vi "Gyro Acc Dec Fwd Dis WIND.vi"(4 "Stop rotation":i32=1200, 6 "Ini. Degrees":sgl, 7 "Motor":cluster{"Port":T2, "Port":T2}={"Port"=1, "Port"=2} {"Port" items=["Port A", "Port B", "Port C", "Port D"]; "Port" items=["Port A", "Port B", "Port C", "Port D"]}, 8 "Threshold to De-acc":i32=1000, 9 "De-acc":i32=40, 10 "Acc":i32=80, 11 "EV3 in":T1) -> (3 "EV3 out":T1)   [LabVIEW 2016]
uses:
  <vilib>/NXT/Block Support/NXT_OutputPort.ctl
  <vilib>/NXT/Subs/LVHSConnector.ctl
  <vilib>/NXT/LegoClasses/BrickReference/BrickReference.lvclass
  <vilib>/NXT/Block Support/NXT_InputPort.ctl
  <vilib>/NXT/NXTIO Xnodes/NXTIONodeSubVIs/LEGOResetMotors.vi
  <vilib>/NXT/Dual Mode Library/Motors/Rotation.vi
  <vilib>/NXT/Dual Mode Library/Sensors/EV3_Gyro_Angle.vi
  <vilib>/NXT/NXTIO Xnodes/NXTIONodeSubVIs/NXTMotorSteeringOn.vi
  <vilib>/NXT/NXTIO Xnodes/NXTIONodeSubVIs/NXTStopMotors.vi
  <vilib>/NXT/Dual Mode Library/Waits/Wait_Num.vi
  <vilib>/NXT/NXTIO Xnodes/NXTIOXNode/NXTIO.xnode
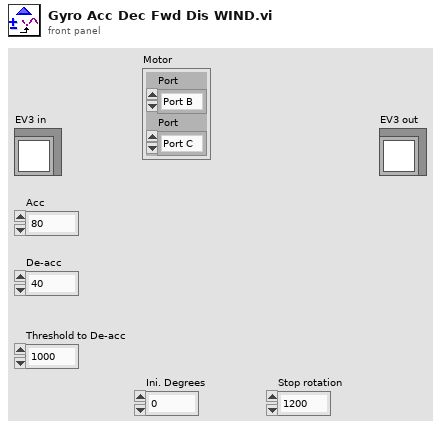
[diagram p1: front panel]
types:
  T1 = typedef "LVHSConnector.ctl" = refnum<class "BrickReference.lvclass">
  T2 = typedef "NXT_OutputPort.ctl" = u8
  T3 = typedef "NXT_InputPort.ctl" = u32
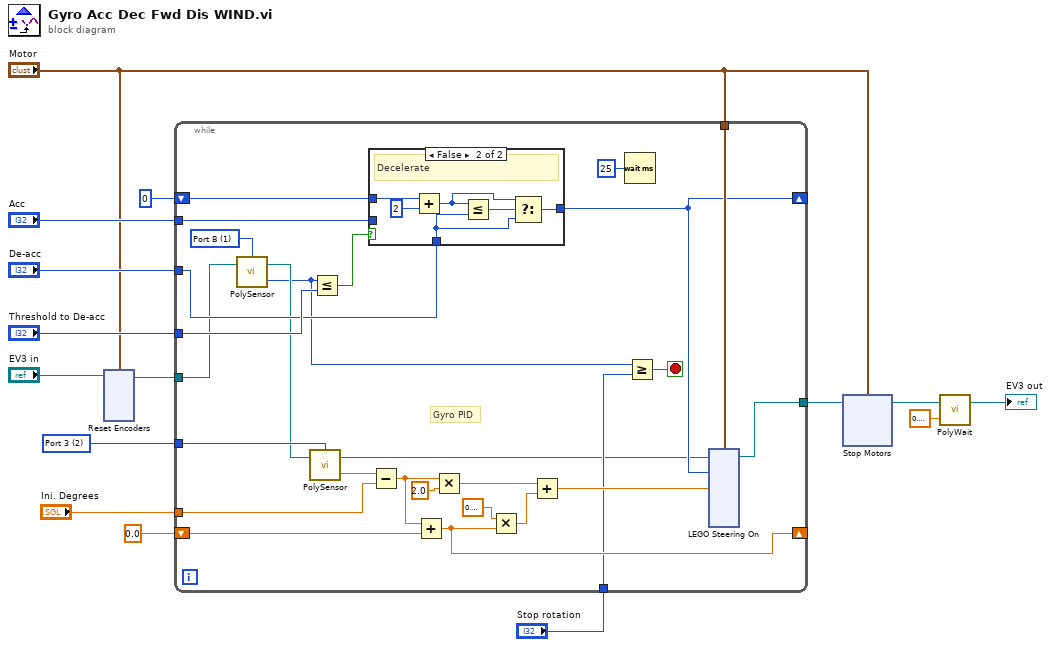
[diagram p0: block diagram]
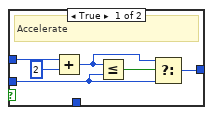
[diagram p2: hidden frame]
diagram:
  w13 = T3 2 items=["Port 1", "Port 2", "Port 3", "Port 4"] ("Port (Gyro)")
  n1 = xnode "Reset Encoders"("Motors"="Motor", "NXT/EV3"="EV3 in") -> ("NXT/EV3"=w10:T1)
  n2 = while {
    tunnel: w10 -> [w23]
    tunnel: w13 -> [w31]
    shift-right: [w39] -> _
    shift-left: sgl 0.0 -> [w40]
    tunnel: "Ini. Degrees" -> [w35]
    tunnel: [w30] -> w6
    tunnel: "Motor" -> [w33]
    shift-right: [w20] -> _
    shift-left: 0 -> [w27]
    tunnel: "De-acc" -> [w24]
    tunnel: "Acc" -> [w26]
    tunnel: "Threshold to De-acc" -> [w25]
    tunnel: "Stop rotation" -> [w17]
    stop <- w19 stop-if-true
    w32 = T2 1 items=["Port A", "Port B", "Port C", "Port D"] ("Port (Port A)")
    # "Gyro PID"
    n3 = call-poly <vilib>:"PolySensor.vi"("NXT/EV3"=w23, "Port (Port A)"=w32) -> ("Angle of Rotation"=w18:i32, "NXT/EV3"=w22:T1)  [unwired: 1 in]
    n4 = call-poly <vilib>:"PolySensor.vi"("NXT/EV3"=w22, "Port (Port 1)"=w31) -> ("Degrees"=w42:sgl, "NXT/EV3"=w16:T1)  [unwired: 1 in]
    n5 = Less Or Equal?(x=w18, y=w25) -> (x <= y?=w21:bool)
    n6 = case shown="False" w21 {
      tunnel: w26 -> [w44 _]
      tunnel: w27 -> [w47 w53]
      tunnel: [w43 w50] -> w20
      tunnel: w24 -> [_ w49]
      frame True {
        # "Accelerate"
        n7 = Add(x=w47, y=2) -> (x+y=w45:i32)
        n8 = Less Or Equal?(x=w45, y=w44) -> (x <= y?=w46:bool)
        n9 = Select(t=w45, s=w46, f=w44) -> (s? t:f=w43:i32)
      }
      frame False {
        # "Decelerate"
        n10 = Add(x=w53, y=2) -> (x+y=w51:i32)
        n11 = Less Or Equal?(x=w51, y=w49) -> (x <= y?=w52:bool)
        n12 = Select(t=w51, s=w52, f=w49) -> (s? t:f=w50:i32)
      }
    }
    n13 = Subtract(x=w42, y=w35) -> (x-y=w34:sgl)
    n14 = Add(x=w34, y=w40) -> (x+y=w39:sgl)
    n15 = Multiply(x=w34, y=sgl 2.0 ("K_p")) -> (x*y=w37:sgl)
    n16 = Multiply(x=sgl 0.1 ("K_i"), y=w39) -> (x*y=w36:sgl)
    n17 = Add(x=w37, y=w36) -> (x+y=w28:sgl)
    n18 = Wait (ms)(milliseconds to wait=u32 25) -> ()  [unwired: 1 out]
    n19 = Greater Or Equal?(x=w18, y=w17) -> (x >= y?=w19:bool)
    n20 = xnode "LEGO Steering On"("Steering 1"=w28, "Power 1"=w20, "Motors"=w33, "NXT/EV3"=w16) -> ("NXT/EV3"=w30:T1)
  }
  n21 = xnode "Stop Motors"("Motors"="Motor", "NXT/EV3"=w6) -> ("NXT/EV3"=w4:T1)
  n22 = call-poly <vilib>:"PolyWait.vi"("Time (1 sec)"=sgl 0.2, "NXT/EV3"=w4) -> ("NXT/EV3"=→"EV3 out":T1)  [unwired: 2 in]
